vi "Button_handling.vi"(7 "connect":bool, 10 "Z_HSwitch":bool, 11 "Z_Source":T2=enum."local disabled") -> (3 "Z_HSwitch_state":T1={"Write"=FALSE, "Z1_ind"=5, "Z1_ind_blinking"=FALSE, "Z_HSwitch_out"=FALSE, "Z_HSwitch_visible"=FALSE, "Z_HSwitch_disabled"=enum."Enabled"})   [LabVIEW 2019, in "Heating.lvlib"]
uses:
  Heating.lvlib
  ctl/Y_source.ctl
  ctl/Z_Hswitch/AutoButton_state.ctl
  Timer Delay/Timers.lvlib
  ctl/Z_Hswitch/Z_Hswitch.xctl
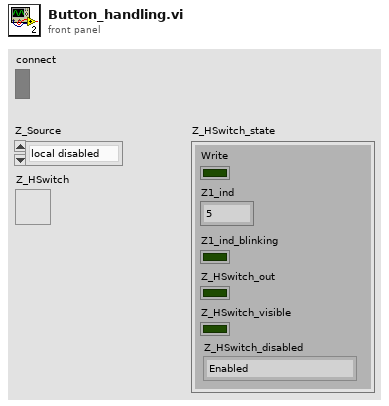
[diagram p1: front panel]
types:
  T1 = cluster{"Write":bool, "Z1_ind":u8, "Z1_ind_blinking":bool, "Z_HSwitch_out":bool, "Z_HSwitch_visible":bool, "Z_HSwitch_disabled":enum8{"Enabled", "Disabled", "Disabled and Grayed Out"}}
  T2 = typedef "Heating.lvlib/Y_source.ctl" = enum8{"initialize", "local disabled", "local hand", "hand", "auto", "dist"}
  T3 = cluster{"Write":bool, "Z1_ind visu":u8, "Z1_ind_blinking":bool, "Z_HSwitch_out":bool, "Z_HSwitch_visible":bool, "Z_HSwitch_disabled":enum8{"Enabled", "Disabled", "Disabled and Grayed Out"}}
  T4 = typedef "Heating.lvlib/Z_Hswitch.xctl/AutoButton_state.ctl" = u16
  T5 = enum8{"Enabled", "Disabled", "Disabled and Grayed Out"}
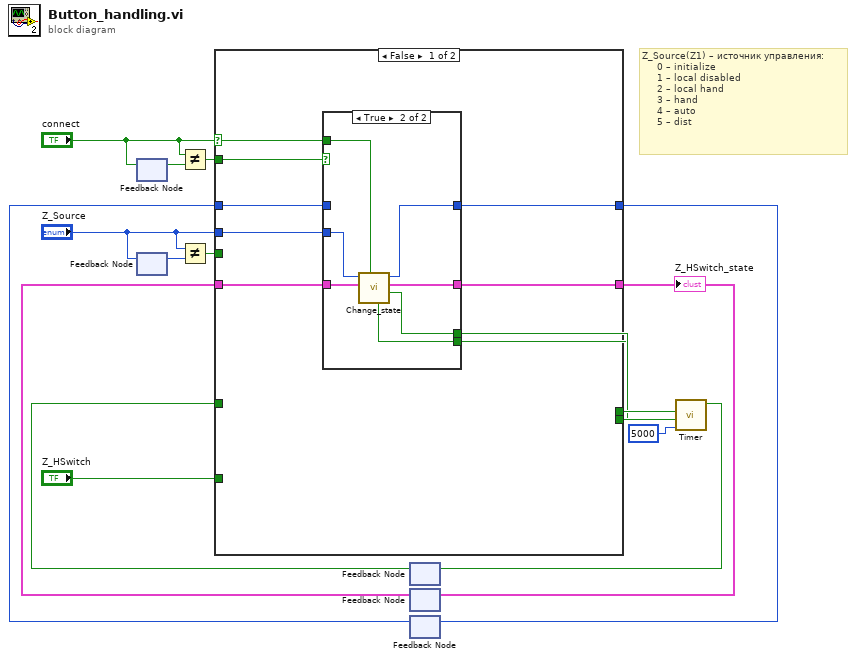
[diagram p0: block diagram]
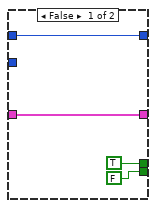
[diagram p2: hidden frame]
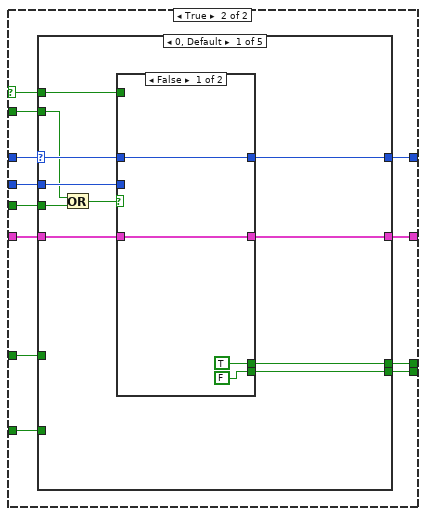
[diagram p3: hidden frame]
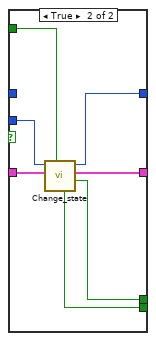
[diagram p4: hidden frame]
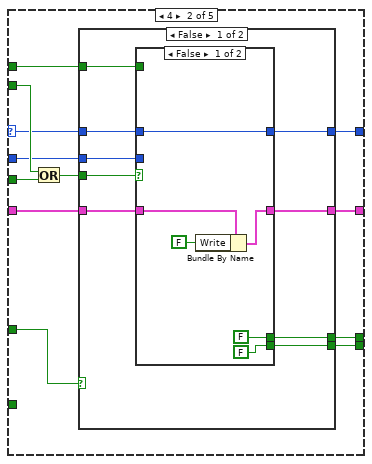
[diagram p5: hidden frame]
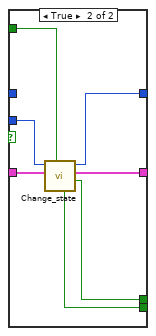
[diagram p6: hidden frame]
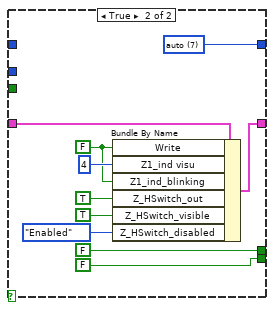
[diagram p7: hidden frame]
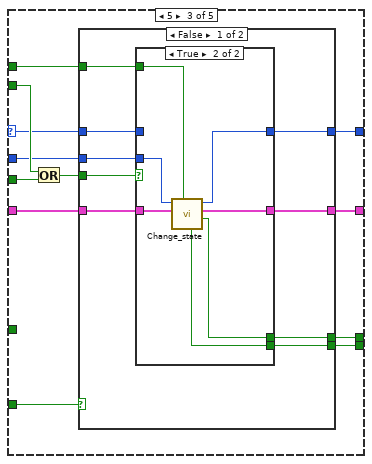
[diagram p8: hidden frame]
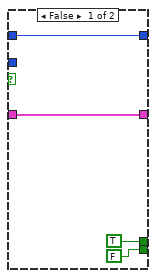
[diagram p9: hidden frame]
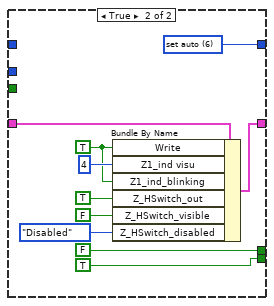
[diagram p10: hidden frame]
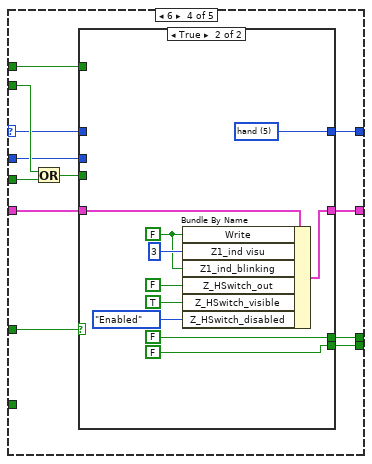
[diagram p11: hidden frame]
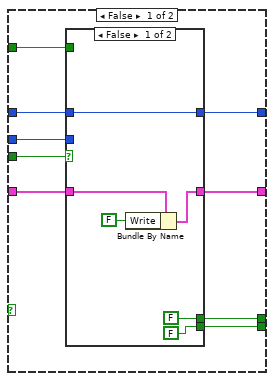
[diagram p12: hidden frame]
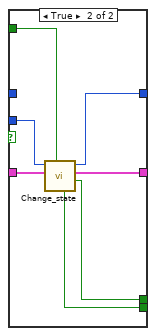
[diagram p13: hidden frame]
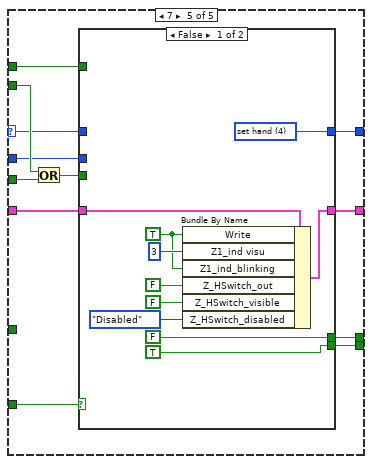
[diagram p14: hidden frame]
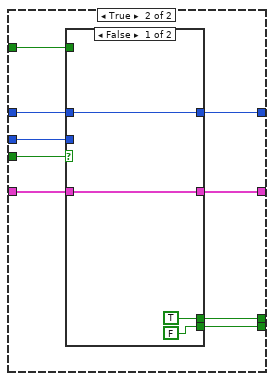
[diagram p15: hidden frame]
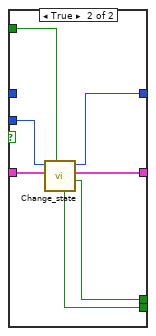
[diagram p16: hidden frame]
diagram:
  # "Z_Source(Z1) – источник управления:\n     0 – initialize\n     1 – local disabled\n     2 – local hand\n     3 – hand\n     4 – аuto\n     5 – dist"
  n1 = feedback #1() -> (w9:bool)  [unwired: 1 in]
  n2 = feedback-in #1("connect") -> ()
  n3 = feedback #2() -> (w12:T2)  [unwired: 1 in]
  n4 = feedback-in #2("Z_Source") -> ()
  n5 = Not Equal?(x="connect", y=w9) -> (x != y?=w7:bool)
  n6 = Not Equal?(x="Z_Source", y=w12) -> (x != y?=w10:bool)
  n7 = feedback #3() -> (w5:bool)  [unwired: 1 in]
  n8 = feedback #4() -> (w3:T3)  [unwired: 1 in]
  n9 = feedback #5() -> (w1:T4)  [unwired: 1 in]
  n10 = case shown="False" "connect" {
    selector: "connect" -> [w17 w39]
    tunnel: [w22 w48] -> w2
    tunnel: w5 -> [_ w47]
    tunnel: w3 -> [w23 w46]
    tunnel: w1 -> [w25 w45]
    tunnel: "Z_HSwitch" -> [_ w44]
    tunnel: "Z_Source" -> [w24 w43]
    tunnel: [w21 w42] -> w4
    tunnel: [w20 w41] -> w14
    tunnel: [w19 w40] -> w13
    tunnel: w10 -> [_ w38]
    tunnel: w7 -> [w18 w37]
    frame False {
      n11 = case shown="True" w18 {
        tunnel: w23 -> [w29 w36]
        tunnel: [w29 w35] -> w21
        tunnel: [TRUE ("reset_timer") w34] -> w20
        tunnel: [FALSE ("load_timer") w33] -> w19
        tunnel: [w26 w32] -> w22
        tunnel: w24 -> [_ w31]
        tunnel: w25 -> [w26 _]
        tunnel: w17 -> [_ w30]
        frame False {
        }
        frame True {
          n12 = call "Change_state.vi"("connect (T)"=w30, "Z_HSwitch_state in"=w36, "Z_Source"=w31) -> ("reset_timer"=w34:bool, "Z_HSwitch_state out"=w35:T3, "Z1_ind_state"=w32:T4, "load_timer"=w33:bool)  [unwired: 5 in]
        }
      }
    }
    frame True {
      n13 = case shown="0, Default" w45 {
        selector: w45 -> [w53 w74 w118 w160 w204]
        tunnel: w44 -> [_ _ w120 _ w206]
        tunnel: [w54 w80 w124 w166 w210] -> w48
        tunnel: w43 -> [w58 w73 w117 w159 w203]
        tunnel: w47 -> [_ w76 _ w162 _]
        tunnel: [w57 w78 w122 w164 w208] -> w41
        tunnel: [w56 w77 w121 w163 w207] -> w40
        tunnel: [w55 w79 w123 w165 w209] -> w42
        tunnel: w46 -> [w59 w71 w115 w157 w201]
        tunnel: w39 -> [w50 w75 w119 w161 w205]
        tunnel: w38 -> [w51 w81 w125 w167 w211]
        tunnel: w37 -> [w49 w82 w126 w168 w212]
        frame 0, Default {
          # "local hand"
          n14 = Or(x=w49, y=w51) -> (x .or. y?=w52:bool)
          n15 = case shown="False" w52 {
            tunnel: w59 -> [w63 w70]
            tunnel: [w63 w69] -> w55
            tunnel: [TRUE ("reset_timer") w68] -> w57
            tunnel: [FALSE ("load_timer") w67] -> w56
            tunnel: [w60 w66] -> w54
            tunnel: w58 -> [_ w65]
            tunnel: w50 -> [_ w64]
            tunnel: w53 -> [w60 _]
            frame False {
            }
            frame True {
              n16 = call "Change_state.vi"("connect (T)"=w64, "Z_HSwitch_state in"=w70, "Z_Source"=w65) -> ("reset_timer"=w68:bool, "Z_HSwitch_state out"=w69:T3, "Z1_ind_state"=w66:T4, "load_timer"=w67:bool)  [unwired: 5 in]
            }
          }
        }
        frame 4 {
          # "local hand"
          n17 = Or(x=w82, y=w81) -> (x .or. y?=w72:bool)
          n18 = case shown="False" w76 {
            tunnel: w74 -> [w86 _]
            tunnel: [w85 w114] -> w80
            tunnel: [w83 w109] -> w79
            tunnel: w71 -> [w84 w108]
            tunnel: [w88 FALSE ("Z_ASwitch")] -> w78
            tunnel: [w87 FALSE ("Z_ASwitch")] -> w77
            tunnel: w75 -> [w91 _]
            tunnel: w73 -> [w90 _]
            tunnel: w72 -> [w89 _]
            frame False {
              n19 = case shown="False" w89 {
                tunnel: w84 -> [w93 w104]
                tunnel: [w92 w103] -> w83
                tunnel: [FALSE ("reset_timer") w102] -> w88
                tunnel: [FALSE ("load_timer") w101] -> w87
                tunnel: [w95 w100] -> w85
                tunnel: w90 -> [_ w99]
                tunnel: w91 -> [_ w98]
                tunnel: w86 -> [w95 _]
                frame False {
                  n20 = Bundle By Name(cluster=w93, "Write"=FALSE) -> (w92:T3)
                }
                frame True {
                  n21 = call "Change_state.vi"("connect (T)"=w98, "Z_HSwitch_state in"=w104, "Z_Source"=w99) -> ("reset_timer"=w102:bool, "Z_HSwitch_state out"=w103:T3, "Z1_ind_state"=w100:T4, "load_timer"=w101:bool)  [unwired: 5 in]
                }
              }
            }
            frame True {
              w111 = FALSE ("Z_ASwitch")
              w114 = T4 7 items=["init", "not connect", "local disabled", "local hand", "set hand", "hand", "set auto", "auto", "dist"] ("f 3")
              n22 = Bundle By Name(cluster=w108, "Write"=w111, "Z1_ind visu"=u8 4, "Z1_ind_blinking"=w111, "Z_HSwitch_out"=TRUE ("Z_ASwitch"), "Z_HSwitch_visible"=TRUE ("Z_ASwitch"), "Z_HSwitch_disabled"=T5."Enabled" ("Disabled")) -> (w109:T3)
            }
          }
        }
        frame 5 {
          # "local hand"
          n23 = Or(x=w126, y=w125) -> (x .or. y?=w116:bool)
          n24 = case shown="False" w120 {
            tunnel: w118 -> [w128 _]
            tunnel: [w127 w156] -> w124
            tunnel: [w129 w151] -> w123
            tunnel: w115 -> [w130 w150]
            tunnel: [w132 FALSE ("Z_ASwitch")] -> w122
            tunnel: [w131 TRUE ("Z_ASwitch")] -> w121
            tunnel: w119 -> [w135 _]
            tunnel: w117 -> [w134 _]
            tunnel: w116 -> [w133 _]
            frame False {
              n25 = case shown="True" w133 {
                tunnel: w130 -> [w139 w146]
                tunnel: [w139 w145] -> w129
                tunnel: [TRUE ("reset_timer") w144] -> w132
                tunnel: [FALSE ("load_timer") w143] -> w131
                tunnel: [w136 w142] -> w127
                tunnel: w134 -> [_ w141]
                tunnel: w135 -> [_ w140]
                tunnel: w128 -> [w136 _]
                frame False {
                }
                frame True {
                  n26 = call "Change_state.vi"("connect (T)"=w140, "Z_HSwitch_state in"=w146, "Z_Source"=w141) -> ("reset_timer"=w144:bool, "Z_HSwitch_state out"=w145:T3, "Z1_ind_state"=w142:T4, "load_timer"=w143:bool)  [unwired: 5 in]
                }
              }
            }
            frame True {
              w153 = TRUE ("Z_ASwitch")
              w156 = T4 6 items=["init", "not connect", "local disabled", "local hand", "set hand", "hand", "set auto", "auto", "dist"] ("f 3")
              n27 = Bundle By Name(cluster=w150, "Write"=w153, "Z1_ind visu"=u8 4, "Z1_ind_blinking"=w153, "Z_HSwitch_out"=TRUE ("Z_ASwitch"), "Z_HSwitch_visible"=FALSE ("Z_ASwitch"), "Z_HSwitch_disabled"=T5."Disabled" ("Disabled")) -> (w151:T3)
            }
          }
        }
        frame 6 {
          # "local hand"
          n28 = Or(x=w168, y=w167) -> (x .or. y?=w158:bool)
          n29 = case shown="True" w162 {
            tunnel: w160 -> [w172 _]
            tunnel: [w171 w200] -> w166
            tunnel: [w169 w195] -> w165
            tunnel: w157 -> [w170 w194]
            tunnel: [w174 FALSE ("Z_ASwitch")] -> w164
            tunnel: [w173 FALSE ("Z_ASwitch")] -> w163
            tunnel: w161 -> [w177 _]
            tunnel: w159 -> [w176 _]
            tunnel: w158 -> [w175 _]
            frame False {
              n30 = case shown="False" w175 {
                tunnel: w170 -> [w179 w190]
                tunnel: [w178 w189] -> w169
                tunnel: [FALSE ("reset_timer") w188] -> w174
                tunnel: [FALSE ("load_timer") w187] -> w173
                tunnel: [w181 w186] -> w171
                tunnel: w176 -> [_ w185]
                tunnel: w177 -> [_ w184]
                tunnel: w172 -> [w181 _]
                frame False {
                  n31 = Bundle By Name(cluster=w179, "Write"=FALSE) -> (w178:T3)
                }
                frame True {
                  n32 = call "Change_state.vi"("connect (T)"=w184, "Z_HSwitch_state in"=w190, "Z_Source"=w185) -> ("reset_timer"=w188:bool, "Z_HSwitch_state out"=w189:T3, "Z1_ind_state"=w186:T4, "load_timer"=w187:bool)  [unwired: 5 in]
                }
              }
            }
            frame True {
              w197 = FALSE ("Z_ASwitch")
              w200 = T4 5 items=["init", "not connect", "local disabled", "local hand", "set hand", "hand", "set auto", "auto", "dist"] ("f 3")
              n33 = Bundle By Name(cluster=w194, "Write"=w197, "Z1_ind visu"=u8 3, "Z1_ind_blinking"=w197, "Z_HSwitch_out"=FALSE ("Z_ASwitch"), "Z_HSwitch_visible"=TRUE ("Z_ASwitch"), "Z_HSwitch_disabled"=T5."Enabled" ("Disabled")) -> (w195:T3)
            }
          }
        }
        frame 7 {
          # "local hand"
          n34 = Or(x=w212, y=w211) -> (x .or. y?=w202:bool)
          n35 = case shown="False" w206 {
            tunnel: w204 -> [_ w224]
            tunnel: [w222 w223] -> w210
            tunnel: [w217 w225] -> w209
            tunnel: w201 -> [w216 w226]
            tunnel: [FALSE ("Z_ASwitch") w228] -> w208
            tunnel: [TRUE ("Z_ASwitch") w227] -> w207
            tunnel: w205 -> [_ w231]
            tunnel: w203 -> [_ w230]
            tunnel: w202 -> [_ w229]
            frame False {
              w219 = TRUE ("Z_ASwitch")
              w222 = T4 4 items=["init", "not connect", "local disabled", "local hand", "set hand", "hand", "set auto", "auto", "dist"] ("f 3")
              n36 = Bundle By Name(cluster=w216, "Write"=w219, "Z1_ind visu"=u8 3, "Z1_ind_blinking"=w219, "Z_HSwitch_out"=FALSE ("Z_ASwitch"), "Z_HSwitch_visible"=FALSE ("Z_ASwitch"), "Z_HSwitch_disabled"=T5."Disabled" ("Disabled")) -> (w217:T3)
            }
            frame True {
              n37 = case shown="False" w229 {
                tunnel: w226 -> [w235 w242]
                tunnel: [w235 w241] -> w225
                tunnel: [TRUE ("reset_timer") w240] -> w228
                tunnel: [FALSE ("load_timer") w239] -> w227
                tunnel: [w232 w238] -> w223
                tunnel: w230 -> [_ w237]
                tunnel: w231 -> [_ w236]
                tunnel: w224 -> [w232 _]
                frame False {
                }
                frame True {
                  n38 = call "Change_state.vi"("connect (T)"=w236, "Z_HSwitch_state in"=w242, "Z_Source"=w237) -> ("reset_timer"=w240:bool, "Z_HSwitch_state out"=w241:T3, "Z1_ind_state"=w238:T4, "load_timer"=w239:bool)  [unwired: 5 in]
                }
              }
            }
          }
        }
      }
    }
  }
  "Z_HSwitch_state" <- w4
  n39 = feedback-in #4(w4) -> ()
  n40 = feedback-in #5(w2) -> ()
  n41 = call "Timer.vi"("ms"=5000, "Load (F)"=w13, "Reset (F)"=w14) -> ("End"=w6:bool)  [unwired: 6 in, 1 out]
  n42 = feedback-in #3(w6) -> ()
